vi "Find Node ID.vi"() -> ()   [LabVIEW 2016]
uses:
  <vilib>/CANopenLib/CANOPEN.llb/CANopen SDO Create.vi
  Get Node ID.vi
  <vilib>/CANopenLib/CANOPEN.llb/CANopen SDO Close.vi
panel:
  out "NODE ID":i32
  out "Node ID":u8
  out "error out":errorcluster
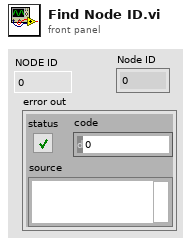
[diagram p1: front panel]
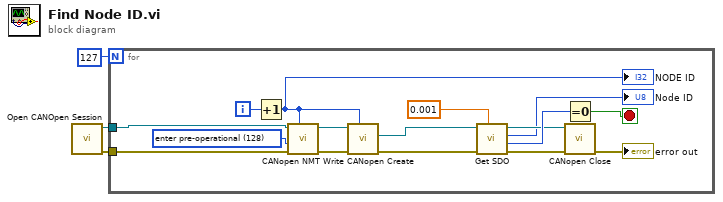
[diagram p0: block diagram]
diagram:
  n1 = call "Open CANOpen Session.vi"() -> ("error out"=w3:errorcluster, "interface object out"=w2:refnum<k20>)  [unwired: 10 in]
  n2 = for {
    N: 127 -> [_]
    tunnel: w3 -> [w19]
    tunnel: w2 -> [w18]
    i -> [w16]
    stop <- w17 stop-if-true
    w4 = u16 128 items=["start remote node"=1, "stop remote node"=2, "enter pre-operational"=128, "reset node"=129, "reset communication"=130] ("command")
    n3 = Increment(x=w16) -> (x+1=w15:i32)
    "NODE ID" <- w15
    n4 = call <vilib>:"CANopen NMT Write.vi"("node-ID (0)"=w15, "error in (no error)"=w19, "command"=w4, "interface object in"=w18) -> ("error out"=w6:errorcluster, "interface object out"=w5:refnum<k20>)  [unwired: 6 in]
    n5 = call-poly <vilib>:"CANopen Create.vi"("node-ID"=w15, "error in (no error)"=w6, "interface object in"=w5) -> ("error out"=w11:errorcluster, "SDO object out"=w10:refnum<k20>)  [unwired: 6 in, 1 out]
    n6 = call-poly "Get SDO.vi"("timeout (1s)"=0.001, "error in (no error)"=w11, "SDO object in"=w10) -> ("error out"=w8:errorcluster, "completion code"=w13:u32, "Node ID"=→"Node ID":u8, "SDO object out"=w9:refnum<k20>)  [unwired: 5 in]
    n7 = Equal To 0?(x=w13) -> (x = 0?=w17:bool)
    n8 = call-poly <vilib>:"CANopen Close.vi"("error in (no error)"=w8, "SDO object in"=w9) -> ("error out"=→"error out":errorcluster)  [unwired: 9 in]
  }
